vi "Translator.File.MatchStrings (Single).vi"(4 "sort? (F)":bool, 7 "group":string, 8 "error in":errorcluster, 9 "label":string, 10 "default value":string, 11 "refnum in":T1) -> (0 "error out":errorcluster, 1 "#added":i32, 2 "value out":string, 3 "refnum out":T1)   [LabVIEW 2019, in "Tools.lvlib"]
uses:
  Tools.lvlib
  <vilib>/Utility/config.llb/Config Data RefNum.ctl
  <vilib>/Utility/config.llb/Read Key (String).vi
  <vilib>/Utility/config.llb/Write Key (String).vi
  <vilib>/Utility/config.llb/NI_LVConfig.lvlib
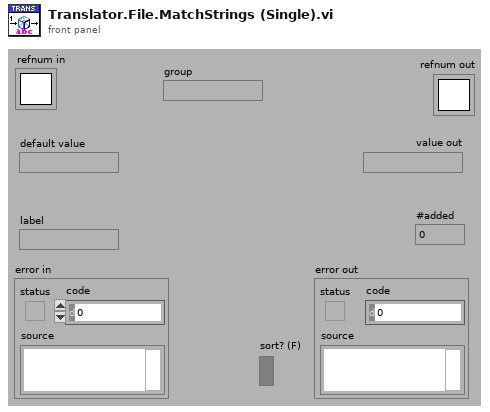
[diagram p1: front panel]
types:
  T1 = typedef "NI_LVConfig.lvlib/Config Data RefNum.ctl" = refnum<k1>
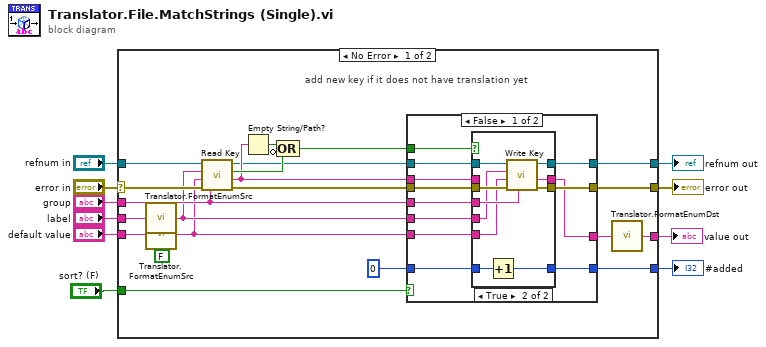
[diagram p0: block diagram]
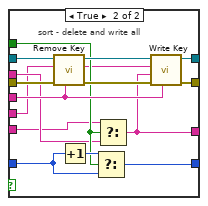
[diagram p3: hidden frame]
diagram:
  n1 = case shown="No Error" "error in" {
    selector: "error in" -> [w29 w73]
    tunnel: "refnum in" -> [w13 w74]
    tunnel: [w19 _] -> w9
    tunnel: [w16 w74] -> w1
    tunnel: [w15 w73] -> w8
    tunnel: [w26 w72] -> w2
    tunnel: "group" -> [w23 _]
    tunnel: "label" -> [w31 _]
    tunnel: "default value" -> [w30 w72]
    tunnel: "sort? (F)" -> [w20 _]
    frame No Error {
      # "add new key if it does not have translation yet"
      n2 = call "Translator.FormatEnumSrc.vi"("text in"=w31) -> ("text out"=w22:string)  [unwired: 1 in]
      n3 = call "Translator.FormatEnumSrc.vi"("text in"=w30, "quotas?(T)"=FALSE) -> ("text out"=w21:string)
      n4 = call-poly <vilib>:"Read Key.vi"("section"=w23, "error in (no error)"=w29, "default value"=w21, "key"=w22, "refnum"=w13) -> ("error out"=w24:errorcluster, "value"=w18:string, "found?"=w27:bool, "refnum out"=w17:T1)  [unwired: 3 in]
      n5 = Empty String/Path?(string/path=w18) -> (empty?=w28:bool)
      n6 = Compound Arithmetic op=OR(w28, invert w27) -> (w12:bool)
      n7 = case shown="False" w20 {
        tunnel: w24 -> [w43 w71]
        tunnel: [w42 w66] -> w15
        tunnel: w17 -> [w41 w70]
        tunnel: [w40 w68] -> w16
        tunnel: w23 -> [w39 w65]
        tunnel: w21 -> [w38 w59]
        tunnel: w12 -> [w37 w61]
        tunnel: w18 -> [w36 w60]
        tunnel: 0 -> [w35 w64]
        tunnel: [w34 w62] -> w19
        tunnel: w22 -> [w33 w57]
        tunnel: [w32 w58] -> w14
        frame False {
          n8 = case shown="True" w37 {
            tunnel: w43 -> [w46 w56]
            tunnel: [w46 w55] -> w42
            tunnel: w41 -> [w47 w54]
            tunnel: [w47 w53] -> w40
            tunnel: w39 -> [_ w52]
            tunnel: w38 -> [_ w48]
            tunnel: w36 -> [w45 _]
            tunnel: w33 -> [_ w51]
            tunnel: [w45 w48] -> w32
            tunnel: w35 -> [w44 w50]
            tunnel: [w44 w49] -> w34
            frame False {
            }
            frame True {
              n9 = Increment(x=w50) -> (x+1=w49:i32)
              n10 = call-poly <vilib>:"Write Key.vi"("section"=w52, "error in (no error)"=w56, "value"=w48, "key"=w51, "refnum"=w54) -> ("error out"=w55:errorcluster, "refnum out"=w53:T1)  [unwired: 4 in, 1 out]
            }
          }
        }
        frame True {
          # "sort - delete and write all"
          n11 = call <vilib>:"Remove Key.vi"("section"=w65, "error in (no error)"=w71, "key"=w57, "refnum"=w70) -> ("error out"=w67:errorcluster, "refnum out"=w69:T1)  [unwired: 5 in, 1 out]
          n12 = Increment(x=w64) -> (x+1=w63:i32)
          n13 = Select(t=w63, s=w61, f=w64) -> (s? t:f=w62:i32)
          n14 = Select(t=w59, s=w61, f=w60) -> (s? t:f=w58:string)
          n15 = call-poly <vilib>:"Write Key.vi"("section"=w65, "error in (no error)"=w67, "value"=w58, "key"=w57, "refnum"=w69) -> ("error out"=w66:errorcluster, "refnum out"=w68:T1)  [unwired: 4 in, 1 out]
        }
      }
      n16 = call "Translator.FormatEnumDst.vi"("text in"=w14) -> ("text out"=w26:string)
    }
    frame Error {
    }
  }
  "#added" <- w9
  "refnum out" <- w1
  "error out" <- w8
  "value out" <- w2
